vi "ConvertCalculateFormatElementsToItemList.vi"(11 "Calculate Format Elements":T1[](array[typedef])) -> (3 "Item List":string)   [LabVIEW 2012, in "Keithley-6482.lvlib"]
uses:
  Public/Controls/CalculateFormatElement.ctl
  Keithley-6482.lvlib
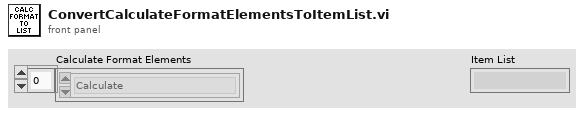
[diagram p1: front panel]
types:
  T1 = typedef "Keithley-6482.lvlib/CalculateFormatElement.ctl" = enum16{"Calculate", "Time", "Status"}
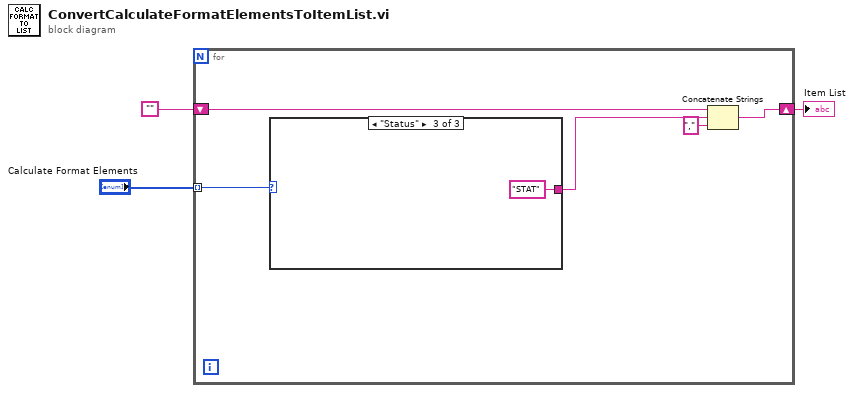
[diagram p0: block diagram]
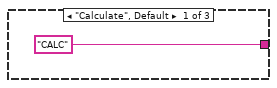
[diagram p2: hidden frame]
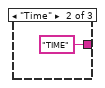
[diagram p3: hidden frame]
diagram:
  n1 = for {
    tunnel: "Calculate Format Elements" -> [w6] mode=indexing
    shift-right: [w7] -> w1
    shift-left: "" -> [w8]
    n2 = case shown="\"Status\"" w6 {
      tunnel: ["CALC" "TIME" "STAT"] -> w5
      frame "Calculate", Default {
      }
      frame "Time" {
      }
      frame "Status" {
      }
    }
    n3 = Concatenate Strings(w8, w5, "," ("string")) -> (w7:string)
  }
  "Item List" <- w1
